vi "FPGA_init_merFISH.vi"(6 "queue FPGA IN":refnum<queue>, 7 "FPGA VI Reference in":refnum<k20>, 8 "error in":errorcluster, 10 "variant":variant, 11 "Measuring QPD":bool) -> (0 "error out":errorcluster, 4 "queue FPGA OUT":refnum<queue>, 5 "FPGA VI Reference Out":refnum<k20>)   [LabVIEW 2015]
uses:
  CONTROLS/Q_FPGA_element.ctl
  <vilib>/FPGAPlugInAG/Dynamic/niLvFpga_Reset_Dynamic.vi
  <vilib>/FPGAPlugInAG/Dynamic/niLvFpga_Close_Dynamic.vi
  <vilib>/FPGAPlugInAG/PCIe-7841R/niLvFpga_Open_PCIe-7841R.vi
  <vilib>/rvi/interface/common/dynamic/niFpgaDynamicAddResources.vi
  <vilib>/FPGAPlugInAG/Dynamic/niLvFpga_Abort_Dynamic.vi
  <vilib>/Utility/error.llb/Error Cluster From Error Code.vi
  <vilib>/rvi/errors/niLvFpgaAdjustHostInterfaceError.vi
  <vilib>/FPGAPlugInAG/Dynamic/niLvFpga_Run_Dynamic.vi
  GLOBAL/Global_FPGA.vi
  <vilib>/rvi/interface/nirviMethod/nirviMethod.xnode
  <vilib>/rvi/interface/nirviCloseFPGA/nirviCloseFPGA.xnode
  <vilib>/rvi/interface/nirviOpenFPGA/nirviOpenFPGA.xnode
  FPGA/FPGA Bitfiles/FPGAv0_FPGATarget_FPGAmerFISHtrigg_IvsmFeOu1pU.lvbitx
  <vilib>/rvi/interface/nirviReadWriteControl/nirviReadWriteControl.xnode
  NiFpgaLv.dll
  <vilib>/rvi/interface/Simulation/niFpgaSimulationCallBeginRW.vi
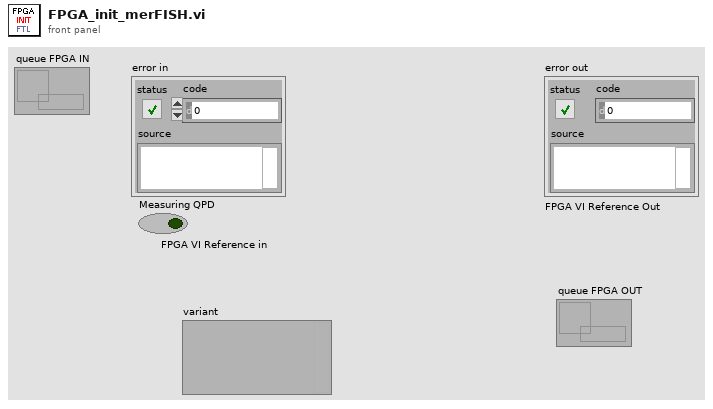
[diagram p1: front panel]
types:
  T1 = typedef "Q_FPGA_element.ctl" = cluster{"variant":variant, "Instruction":enum16{"FPGA_idle", "FPGA_initialize", "FPGA_error", "FPGA_security_stop", "FPGA_laser", "FPGA_start_stop_measure_QPD", "FPGA_measure_QPD", "FPGA_measure_QPD_noise", "FPGA_stop_measure_QPD", "FPGA_init_autofocus", "FPGA_init_single_scan", "FPGA_stop_single_scan", "FPGA_init_merFISH", "FPGA_measure_QPD_merFISH", "FPGA_init_scan_merFISH", "FPGA_scan_merFISH", "FPGA_close_merFISH", "FPGA_stop"}}
  T2 = cluster{"N laser lines":i32, "N Z positions":i32, "Laser lines":i32[], "Laser power":sgl[]}
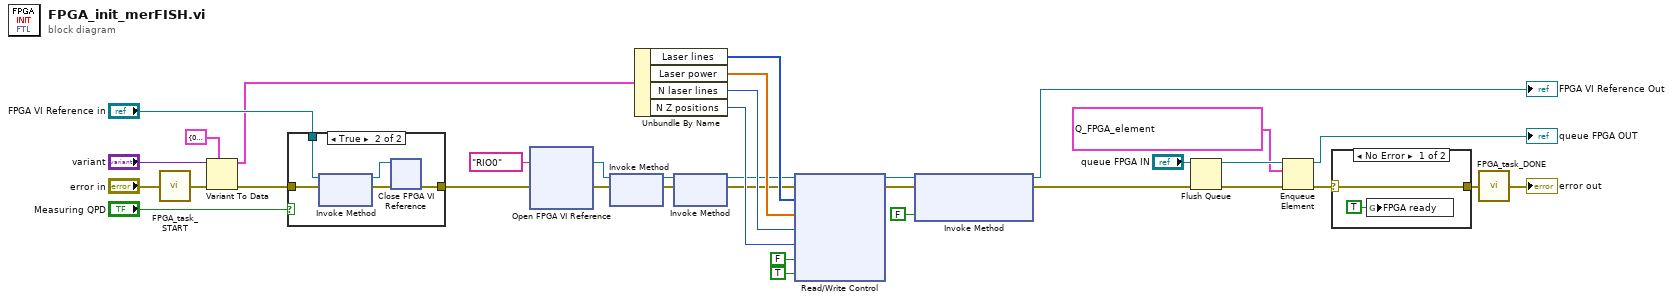
[diagram p0: block diagram]
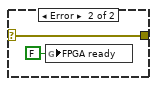
[diagram p3: hidden frame]
diagram:
  n1 = call "FPGA_task_START.vi"("error in"="error in") -> ("error out"=w25:errorcluster)
  n2 = Variant To Data(error in=w25, type=T2 {"N laser lines"=0, "N Z positions"=0, "Laser lines"=[0, 0, 0, 0, 0], "Laser power"=[0.0, 0.0, 0.0, 0.0, 0.0]} ("FPGA cluster"), Variant="variant") -> (data=w17:T2, error out=w26:errorcluster)
  n3 = case shown="True" "Measuring QPD" {
    tunnel: w26 -> [w36 w41]
    tunnel: "FPGA VI Reference in" -> [_ w40]
    tunnel: [w36 w37] -> w20
    frame False {
    }
    frame True {
      n4 = xnode "Invoke Method"("FPGA VI Reference In"=w40, "error in"=w41) -> ("FPGA VI Reference Out"=w38:refnum<k20>, "error out"=w39:errorcluster)
      n5 = xnode "Close FPGA VI Reference"("FPGA VI Reference In"=w38, "error in"=w39) -> ("error out"=w37:errorcluster)
    }
  }
  n6 = xnode "Open FPGA VI Reference"("error in"=w20, "resource name"=tag "RIO0") -> ("FPGA VI Reference Out"=w7:refnum<k20>, "error out"=w8:errorcluster)
  n7 = xnode "Invoke Method"("FPGA VI Reference In"=w7, "error in"=w8) -> ("FPGA VI Reference Out"=w6:refnum<k20>, "error out"=w5:errorcluster)
  n8 = Unbundle By Name(w17) -> ("Laser lines"=w32:i32[], "Laser power"=w33:sgl[], "N laser lines"=w34:i32, "N Z positions"=w35:i32)
  n9 = xnode "Invoke Method"("FPGA VI Reference In"=w6, "error in"=w5) -> ("FPGA VI Reference Out"=w4:refnum<k20>, "error out"=w3:errorcluster)
  n10 = xnode "Read/Write Control"("FPGA VI Reference In"=w4, "error in"=w3, "Laser lines"=w32, "Laser power"=w33, "N laser lines"=w34, "N Z positions"=w35, "stop"=FALSE, "Reset counter"=TRUE) -> ("FPGA VI Reference Out"=w29:refnum<k20>, "error out"=w30:errorcluster)
  n11 = xnode "Invoke Method"("FPGA VI Reference In"=w29, "error in"=w30, "Wait Until Done (F)"=FALSE) -> ("FPGA VI Reference Out"=→"FPGA VI Reference Out":refnum<k20>, "error out"=w13:errorcluster)
  n12 = Flush Queue(queue="queue FPGA IN", error in (no error)=w13) -> (queue out=w15:refnum<queue>, error out=w14:errorcluster)  [unwired: 1 out]
  n13 = Enqueue Element(queue=w15, element=T1 {"variant"=variant, "Instruction"=enum."FPGA_measure_QPD_merFISH"}, error in (no error)=w14) -> (queue out=→"queue FPGA OUT":refnum<queue>, error out=w10:errorcluster)  [unwired: 1 in, 1 out]
  n14 = case shown="No Error" w10 {
    selector: w10 -> [w42 w44]
    tunnel: [w42 w44] -> w19
    frame No Error {
      n15 = global write "Global_FPGA.vi" "FPGA ready"(TRUE ("FPGA ready")) -> ()
    }
    frame Error {
      n16 = global write "Global_FPGA.vi" "FPGA ready"(FALSE ("FPGA ready")) -> ()
    }
  }
  n17 = call "FPGA_task_DONE.vi"("error in"=w19) -> ("error out"=→"error out":errorcluster)
